vi "FRCts20_WebMethods_Convert_SingleEvent.vi"(8 "error in (no error)":errorcluster, 11 "Event Out":T1) -> (0 "error out":errorcluster, 3 "Event":T2)   [LabVIEW 2012, in "FRCts20_WebMethods.lvlib"]
uses:
  FRCts20_WebMethods.lvlib
  ESP Engine/source/VI Source/TypeDefs/FRCts20_EspEngine_Event.ctl
  Web Method Public Interface/FRCts20_WebMethods_ctl_singleEvent.ctl
  Web Method Public Interface/FRCts20_WebMethods_ctl_teamIdentifier.ctl
  Backend/source/VI Source/FRCts20_Backend_API/FRCts20_Backend_API_Event.ctl
  ESP Engine/source/VI Source/FRCts20_EspEngine.lvlib
  Backend/source/VI Source/FRCts20_Backend_API/FRCts20_Backend_API.lvlib
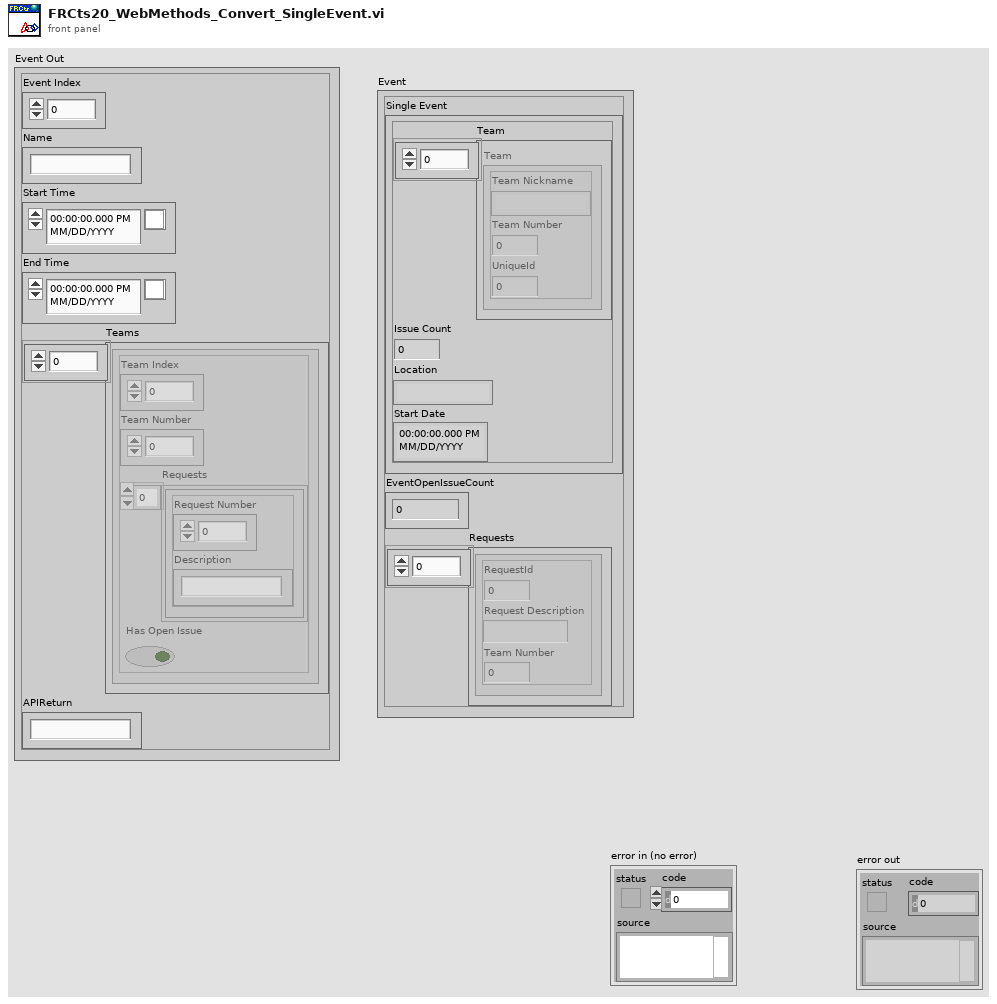
[diagram p1: front panel]
types:
  T1 = typedef "FRCts20_Backend_API.lvlib/FRCts20_Backend_API_Event.ctl" = cluster{"Event Index":u32, "Name":string, "Start Time":timestamp, "End Time":timestamp, "Teams":cluster{"Team Index":u32, "Team Number":u32, "Requests":cluster{"Request Number":u32, "Description":string}[], "Has Open Issue":bool}[], "APIReturn":string}
  T2 = typedef "FRCts20_EspEngine.lvlib/FRCts20_EspEngine_Event.ctl" = cluster{"Single Event":T3, "EventOpenIssueCount":i16, "Requests":cluster{"RequestId":i32, "Request Description":string, "Team Number":i32}[]}
  T3 = typedef "FRCts20_WebMethods.lvlib/FRCts20_WebMethods_ctl_singleEvent.ctl" = cluster{"Team":T4[], "Issue Count":i32, "Location":string, "Start Date ":timestamp}
  T4 = typedef "FRCts20_WebMethods.lvlib/FRCts20_WebMethods_ctl_teamIdentifier.ctl" = cluster{"Team Nickname":string, "Team Number ":u32, "UniqueId":u32}
  T5 = cluster{"RequestId":i32, "Request Description":string, "Team Number":i32}
  T6 = cluster{"Team Index":u32, "Team Number":u32, "Requests":cluster{"Request Number":u32, "Description":string}[], "Has Open Issue":bool}[]
  T7 = cluster{"Request Number":u32, "Description":string}[]
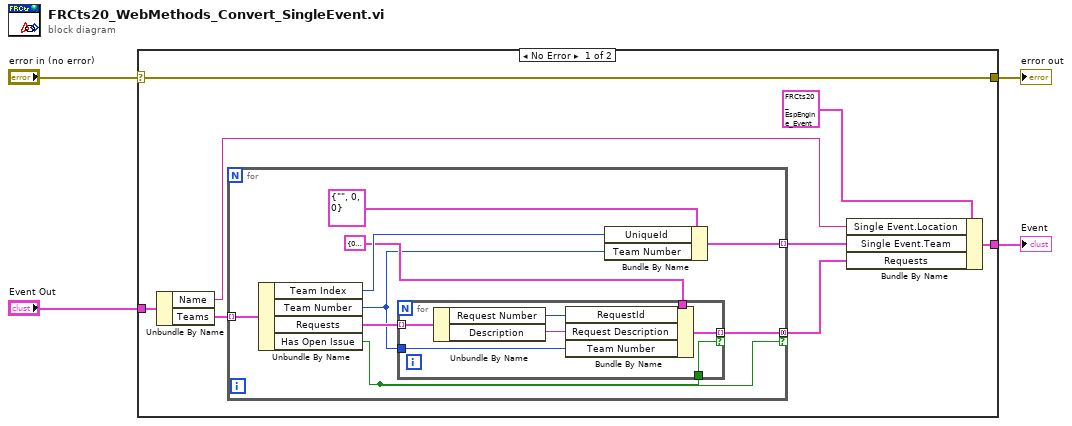
[diagram p0: block diagram]
diagram:
  n1 = case shown="No Error" "error in (no error)" {
    selector: "error in (no error)" -> [w5 w29]
    tunnel: [w5 w29] -> w4
    tunnel: "Event Out" -> [w7 _]
    tunnel: [w6 _] -> w1
    frame No Error {
      n2 = Unbundle By Name(w7) -> ("Name"=w11:string, "Teams"=w10:T6)
      n3 = for {
        tunnel: w10 -> [w21] mode=indexing
        tunnel: [w18] -> w9 mode=indexing
        tunnel: [w16] -> w8 mode=concatenating if=w13
        n4 = Unbundle By Name(w21) -> ("Team Index"=w19:u32, "Team Number"=w14:u32, "Requests"=w15:T7, "Has Open Issue"=w13:bool)
        n5 = for {
          tunnel: T5 {"RequestId"=0, "Request Description"="", "Team Number"=0} ("Request") -> [w28]
          tunnel: [w27] -> w16 mode=indexing if=w22
          tunnel: w15 -> [w26] mode=indexing
          tunnel: w14 -> [w23]
          tunnel: w13 -> [w22]
          n6 = Unbundle By Name(w26) -> ("Request Number"=w25:u32, "Description"=w24:string)
          n7 = Bundle By Name(cluster=w28, "RequestId"=w25, "Request Description"=w24, "Team Number"=w23) -> (w27:T5)
        }
        n8 = Bundle By Name(cluster=T4 {"Team Nickname"="", "Team Number "=0, "UniqueId"=0} ("Team"), "UniqueId"=w19, "Team Number"=w14) -> (w18:T4)
      }
      n9 = Bundle By Name(cluster=T2 {"Single Event"={"Team"=[], "Issue Count"=0, "Location"="", "Start Date "=timestamp(0 s since 1904-01-01)}, "EventOpenIssueCount"=0, "Requests"=[]} ("Event"), "Single Event.Location"=w11, "Single Event.Team"=w9, "Requests"=w8) -> (w6:T2)
    }
    frame Error {
    }
  }
  "Event" <- w1
  "error out" <- w4
